vi "logic-train-sample-7-1-TEST-drum-seq.vi"() -> ()   [LabVIEW 2020]
uses:
  <vilib>/Rock Robotics/WPI/ThirdParty/JAS_Junk/TrajLib/Enum/DrumSequence_Step_Enum.ctl
  <vilib>/Rock Robotics/WPI/ThirdParty/JAS_Junk/TrajLib/Trajectory_Library.lvlib
panel:
  out "Error":bool
  out "Seq  Active":bool
  out "Ready":bool
  out "Step Number":T1=enum."Initialize"
  in  "Cancel":bool
  in  "Request\nCapture":bool
  out "Hand_Close":bool
  out "Arm_Extend":bool
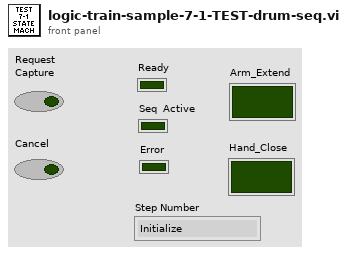
[diagram p1: front panel]
types:
  T1 = typedef "Trajectory_Library.lvlib/DrumSequence_Step_Enum.ctl" = enum16{"Do Nothing", "Step 1", "Step 2", "Step 3", "Step 4", "Step 5", "Step 6", "Step 7", "Step 8", "Step 9", "Step 10", "Step 11", "Step 12", "Step 13", "Step 14", "Step 15", "Step 16", "Step 17", "Step 18", "Step 19", "Step 20", "Step 21", "Step 22", "Step 23", "Step 24", "Step 25", "Step 26", "Step 27", "Step 28", "Step 29", "Step 30", "Step 31", "Step 32", "Cancel", "Initialize", "Error"}
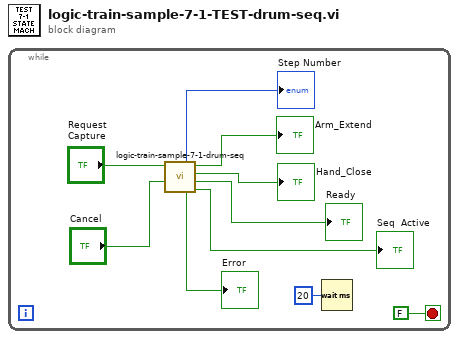
[diagram p0: block diagram]
diagram:
  n1 = while {
    stop <- FALSE stop-if-true
    n2 = call "logic-train-sample-7-1-drum-seq.vi"("Cancel"="Cancel", "Request\nCapture"="Request\nCapture") -> ("Seq  Active"=→"Seq  Active":bool, "Ready"=→"Ready":bool, "Hand_Close"=→"Hand_Close":bool, "Arm_Extend"=→"Arm_Extend":bool, "Error"=→"Error":bool, "Step Number"=→"Step Number":T1)  [unwired: 4 in]
    n3 = Wait (ms)(milliseconds to wait=u32 20) -> ()  [unwired: 1 out]
  }
